vi "Laser Feedback-PD ver2.vi"() -> ()   [LabVIEW 2014]
uses:
  <vilib>/Analysis/baseanly.llb/Mean (DBL).vi
  <vilib>/DAQmx/create/channels.llb/DAQmx Create Channel (AI-Voltage-Basic).vi
  <vilib>/DAQmx/create/channels.llb/DAQmx Create Channel (AO-Voltage-Basic).vi
  <vilib>/DAQmx/configure/timing.llb/DAQmx Timing (Sample Clock).vi
  Main-Stage-Based/(Global) Current handle and LaserPower_YCC.vi
  <vilib>/Analysis/polynomials.llb/Scalar Polynomial Evaluation (DBL).vi
  <vilib>/DAQmx/read.llb/DAQmx Read (Analog 1D DBL 1Chan NSamp).vi
  <vilib>/addons/control/pid/pid.llb/PID (DBL).vi
  <vilib>/DAQmx/write.llb/DAQmx Write (Analog DBL 1Chan 1Samp).vi
  <vilib>/Utility/file.llb/Write To Spreadsheet File (DBL).vi
  <vilib>/Analysis/NI_AALPro.lvlib
  <vilib>/addons/control/pid/NI_PID_pid.lvlib
  <vilib>/Analysis/NI_AALBase.lvlib
panel:
  in  "rate":dbl=9000.0 format="%0.2f"
  in  "physical channels":tag="Dev2/ai19"
  in  "Max voltage (V)":dbl=4.5
  in  "Min voltage (V)":dbl=0.5
  in  "Save feedback data?":bool
  in  "PID gains 2":T1={"proportional gain (Kc)"=0.016099999999999996, "integral time (Ti, min)"=3.100000000000001e-06, "derivative time (Td, min)"=0.0} {"derivative time (Td, min)" format="%#.6g"; "integral time (Ti, min)" format="%#.6g"; "proportional gain (Kc)" format="%#.6g"}
  in  "stop":bool
  out "Photodiode readout (mV)":dbl
  out "Set Laser power (mV)":dbl
  out "AOM (V)":dbl format="%.2f"
  out "Polynomial Coefficients":dbl[](array[numeric])
  in  "Tab Control":T2(tab)
  out "XY Graph":T3(graph)
  out "Waveform Chart":dbl(graph)
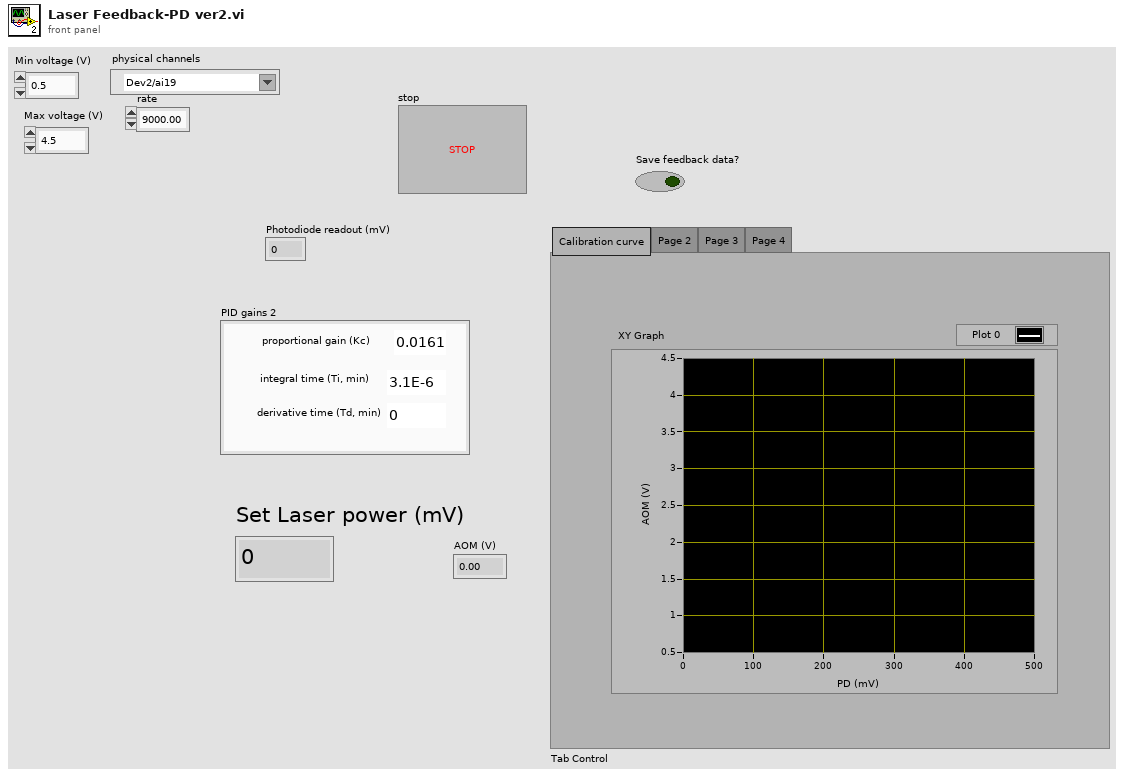
[diagram p1: front panel]
types:
  T1 = cluster{"proportional gain (Kc)":dbl, "integral time (Ti, min)":dbl, "derivative time (Td, min)":dbl}
  T2 = enum32{"Calibration curve", "Page 2", "Page 3", "Page 4"}
  T3 = cluster{"Cal-PD (mV)":dbl[], "Best Polynomial Fit":dbl[]}[]
  T4 = cluster{"Cal-PD (mV)":dbl[], "Cal-AOM (V)":dbl[], "Best Polynomial Fit":dbl[], "Polynomial Coefficients":dbl[]}
  T5 = cluster{"Cal-PD (mV)":dbl[], "Cal-AOM (V)":dbl[]}
  T6 = cluster{"Cal-PD (mV)":dbl[], "Best Polynomial Fit":dbl[]}
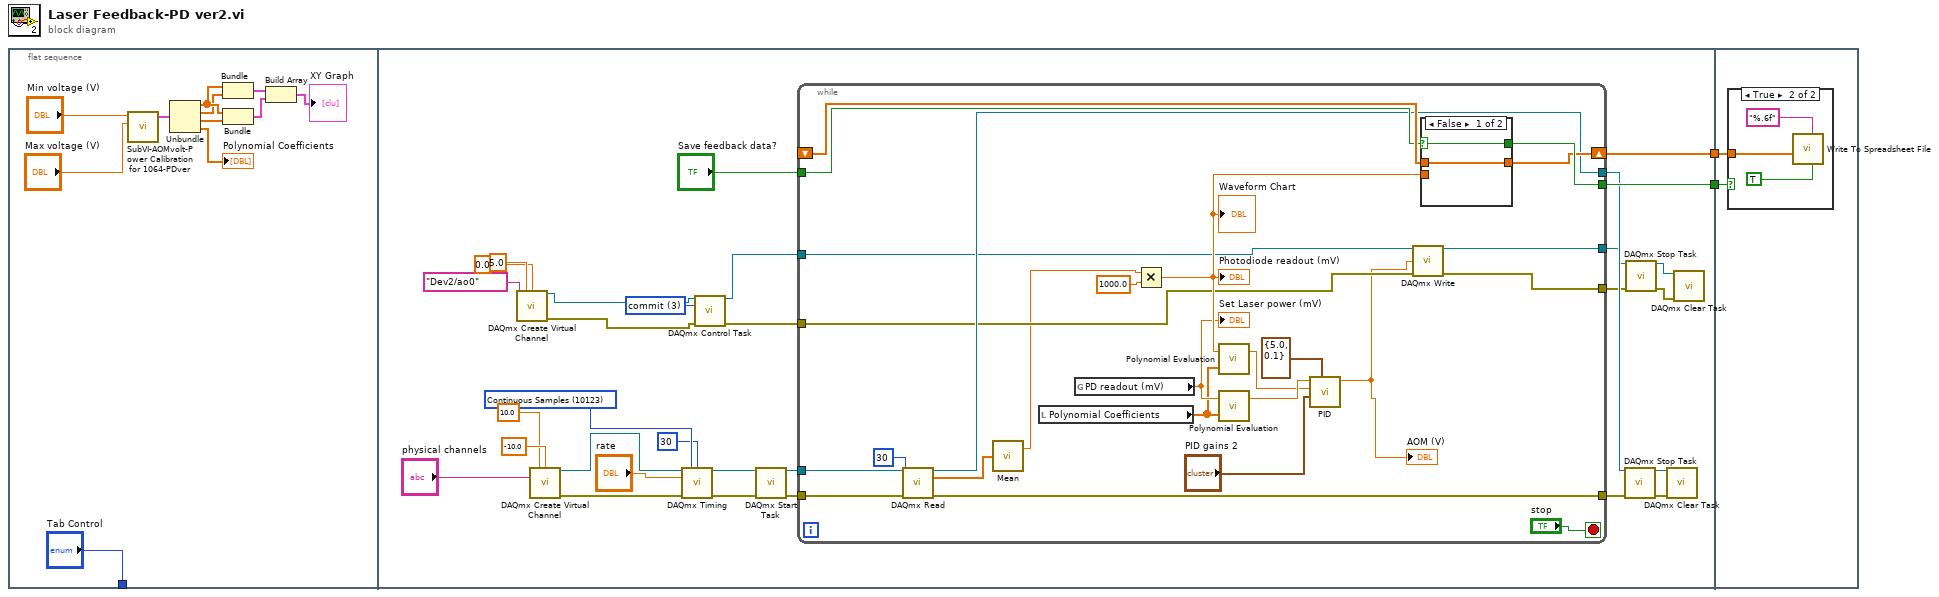
[diagram p0: block diagram]
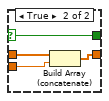
[diagram p2: hidden frame]
diagram:
  n1 = flat-sequence {
    tunnel: ["Tab Control"] -> _
    tunnel: [w43] -> w2
    tunnel: [w42] -> w1
    tunnel: w2 -> [w77]
    tunnel: w1 -> [w76]
    frame #0 {
      n2 = call "SubVI-AOMvolt-Power Calibration for 1064-PDver.vi"("Max voltage (V)"="Max voltage (V)", "Min voltage (V)"="Min voltage (V)") -> ("output cluster"=w13:T4)  [unwired: 3 in, 1 out]
      n3 = Unbundle(w13) -> ("Cal-PD (mV)"=w12:dbl[], "Cal-AOM (V)"=w11:dbl[], "Best Polynomial Fit"=w10:dbl[], "Polynomial Coefficients"=→"Polynomial Coefficients":dbl[])
      n4 = Bundle("Cal-PD (mV)"=w12, "Cal-AOM (V)"=w11) -> (w8:T5)  [unwired: 1 in]
      n5 = Bundle("Cal-PD (mV)"=w12, "Best Polynomial Fit"=w10) -> (w7:T6)  [unwired: 1 in]
      n6 = Build Array(w8, w7) -> (→"XY Graph":T3)
    }
    frame #1 {
      w21 = 3 items=["verify"=2, "reserve"=4, "commit"=3, "unreserve"=5, "abort"=6] ("action")
      w30 = 10123 items=["Finite Samples"=10178, "Continuous Samples"=10123, "Hardware Timed Single Point"=12522] ("sample mode")
      n7 = call-poly <vilib>:"DAQmx Create Virtual Channel.vi"("maximum value"=5.0, "minimum value"=0.0, "physical channels"=tag "Dev2/ao0") -> ("task out"=w23:refnum<k21>, "error out"=w22:errorcluster)  [unwired: 11 in]
      n8 = call-poly <vilib>:"DAQmx Create Virtual Channel.vi"("maximum value"=10.0, "minimum value"=-10.0, "physical channels"="physical channels") -> ("task out"=w41:refnum<k21>, "error out"=w40:errorcluster)  [unwired: 11 in]
      n9 = call-poly <vilib>:"DAQmx Timing.vi"("task/channels in"=w41, "sample mode"=w30, "samples per channel"=30, "rate"="rate", "error in"=w40) -> ("task out"=w39:refnum<k21>, "error out"=w38:errorcluster)  [unwired: 9 in]
      n10 = call <vilib>:"DAQmx Control Task.vi"("task/channels in"=w23, "action"=w21, "error in"=w22) -> ("task out"=w20:refnum<k21>, "error out"=w19:errorcluster)  [unwired: 11 in]
      n11 = call <vilib>:"DAQmx Start Task.vi"("task/channels in"=w39, "error in"=w38) -> ("task out"=w37:refnum<k21>, "error out"=w36:errorcluster)  [unwired: 12 in]
      n12 = while {
        tunnel: [w64] -> w43
        shift-right: [w63] -> w42
        shift-left: _ -> [w62]
        tunnel: "Save feedback data?" -> [w57]
        tunnel: w37 -> [w56]
        tunnel: w36 -> [w55]
        tunnel: [w54] -> w33
        tunnel: [w53] -> w32
        tunnel: w20 -> [w52]
        tunnel: w19 -> [w51]
        tunnel: [w49] -> w18
        tunnel: [w48] -> w17
        stop <- "stop" stop-if-true
        n13 = call-poly <vilib>:"DAQmx Read.vi"("task/channels in"=w56, "number of samples per channel"=30, "error in"=w55) -> ("task out"=w54:refnum<k21>, "data"=w47:dbl[], "error out"=w53:errorcluster)  [unwired: 10 in]
        n14 = call-poly <vilib>:"Mean.vi"("X"=w47) -> ("mean"=w46:dbl)  [unwired: 1 out]
        n15 = local read "Polynomial Coefficients"() -> (w58:dbl[])
        n16 = global read "(Global) Current handle and LaserPower_YCC.vi" "PD readout (mV)"() -> (w59:dbl)
        "Set Laser power (mV)" <- w59
        n17 = Multiply(x=w46, y=1000.0) -> (x*y=w60:dbl)
        "Photodiode readout (mV)" <- w60
        "Waveform Chart" <- w60
        n18 = call-poly <vilib>:"Polynomial Evaluation.vi"("P(x)"=w58, "a"=w60) -> ("P(a)"=w67:dbl)  [unwired: 1 out]
        n19 = call-poly <vilib>:"Polynomial Evaluation.vi"("P(x)"=w58, "a"=w59) -> ("P(a)"=w68:dbl)  [unwired: 1 out]
        n20 = call-poly <vilib>:"PID.vi"("output range"=cluster{"output high":dbl, "output low":dbl} {"output high"=5.0, "output low"=0.1}, "PID gains"="PID gains 2", "process variable"=w67, "setpoint"=w68) -> ("output"=w50:dbl)  [unwired: 6 in, 1 out]
        "AOM (V)" <- w50
        n21 = call-poly <vilib>:"DAQmx Write.vi"("task/channels in"=w52, "data"=w50, "error in"=w51) -> ("task out"=w49:refnum<k21>, "error out"=w48:errorcluster)  [unwired: 10 in, 1 out]
        n22 = case shown="False" w57 {
          selector: w57 -> [w71 w75]
          tunnel: [w71 w75] -> w64
          tunnel: w60 -> [_ w73]
          tunnel: [w70 w72] -> w63
          tunnel: w62 -> [w70 w74]
          frame False {
          }
          frame True {
            n23 = Build Array (concatenate)(w74, w73) -> (w72:dbl[])
          }
        }
      }
      n24 = call <vilib>:"DAQmx Stop Task.vi"("task/channels in"=w33, "error in"=w32) -> ("task out"=w35:refnum<k21>, "error out"=w34:errorcluster)  [unwired: 12 in]
      n25 = call <vilib>:"DAQmx Stop Task.vi"("task/channels in"=w18, "error in"=w17) -> ("task out"=w16:refnum<k21>, "error out"=w15:errorcluster)  [unwired: 12 in]
      n26 = call <vilib>:"DAQmx Clear Task.vi"("task in"=w35, "error in"=w34) -> ()  [unwired: 13 in, 1 out]
      n27 = call <vilib>:"DAQmx Clear Task.vi"("task in"=w16, "error in"=w15) -> ()  [unwired: 13 in, 1 out]
    }
    frame #2 {
      n28 = case shown="True" w77 {
        tunnel: w76 -> [_ w80]
        frame False {
        }
        frame True {
          n29 = call-poly <vilib>:"Write To Spreadsheet File.vi"("transpose? (no:F)"=TRUE, "format (%.3f)"="%.6f", "1D data"=w80) -> ()  [unwired: 5 in, 1 out]
        }
      }
    }
  }
